vi "Build.vi"(9 "XYZTheta":dbl[](array[numeric]), 10 "Pattern Coordinates":dbl[][](array[numeric]), 11 "CAD Dispense in":refnum<class "CAD Dispense.lvclass">) -> (1 "Starting Coordinates":dbl[](array[numeric]), 3 "CAD Dispense out":refnum<class "CAD Dispense.lvclass">)   [LabVIEW 2016, in "CAD Dispense.lvclass"]
uses:
  CAD Dispense.lvclass
  CAD Dispense.lvclass/CAD Dispense.ctl
  <vilib>/Analysis/coordinate.llb/2D Cartesian Coordinate Rotation (Scalar).vi
  <vilib>/Analysis/NI_AALPro.lvlib
panel:
  out "Array 3":dbl[][](array[numeric])
  out "size(s) 2":i32
  out "size(s)":i32
  out "startXY,endXY":dbl[][](array[numeric])
  out "center portion":dbl[][](array[numeric])
  out "Array 2":dbl[][](array[numeric])
  out "Array":dbl[][](array[numeric])
  out "array w/ subset deleted 2":T1(array[cluster])
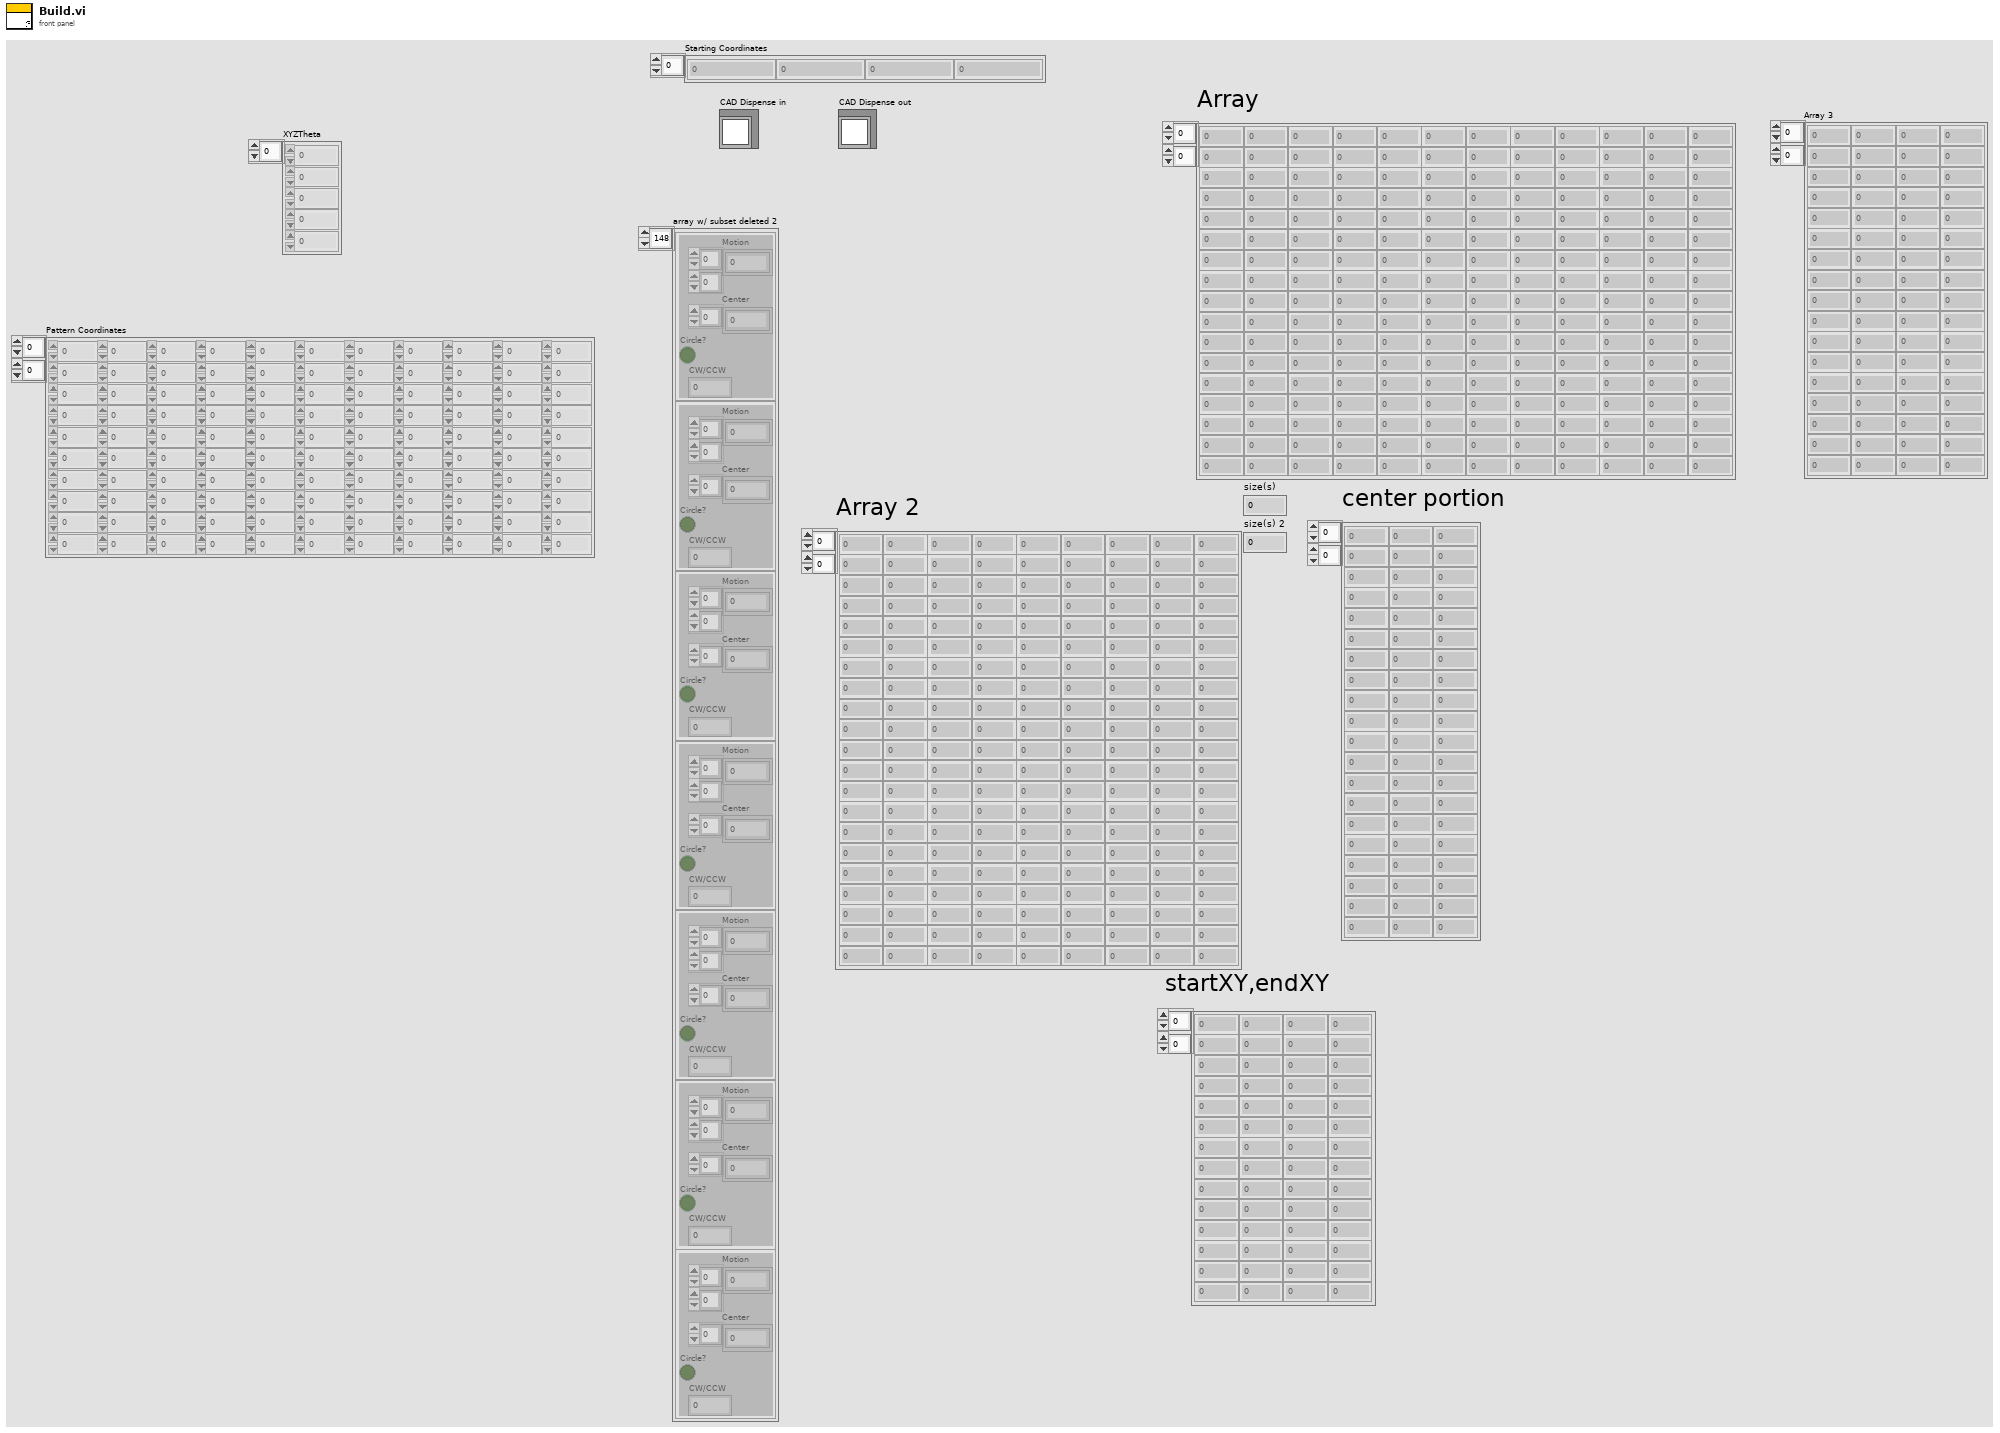
[diagram p1: front panel]
types:
  T1 = cluster{"Motion":dbl[][], "Center":dbl[], "Circle?":bool, "CW/CCW":dbl}[]
  T2 = cluster{"Motion":dbl[][], "Center":dbl[], "Circle?":bool, "CW/CCW":dbl}
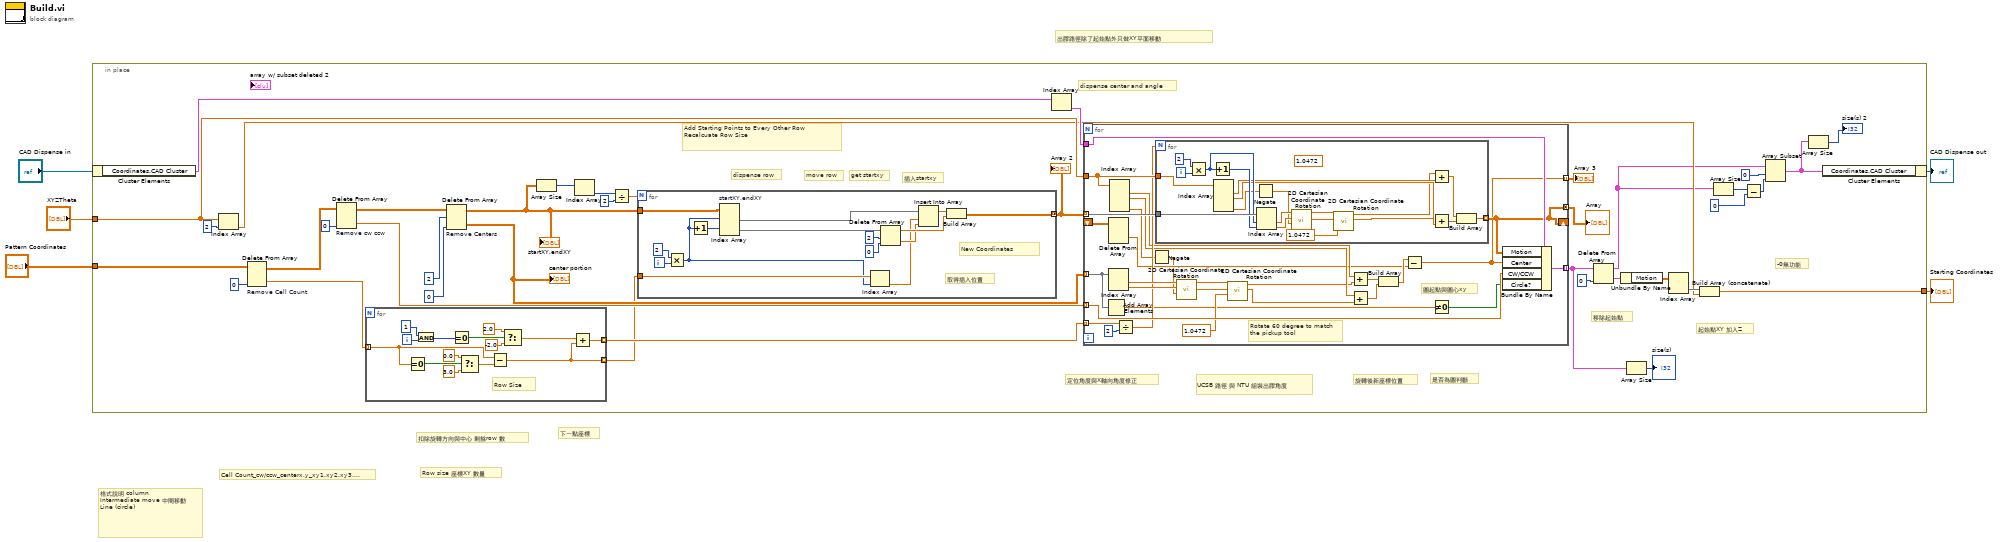
[diagram p0: block diagram]
diagram:
  # "出膠路徑除了起始點外只做XY平面移動"
  # "下一點座標"
  # "Cell Count_cw/ccw_centerx,y_xy1,xy2,xy3,..."
  # "格式說明 column\nIntermediate move 中間移動\nLine (circle)"
  # "扣除旋轉方向與中心 剩餘row 數"
  # "Row size 座標XY 數量"
  n1 = in-place {
    in-place-border: "XYZTheta" -> [w20]
    in-place-border: "Pattern Coordinates" -> [w31]
    in-place-border: [w17] -> w3
    # "-0無功能"
    # "起始點XY 加入Z"
    # "移除起始點"
    # "是否為圓判斷"
    # "旋轉後新座標位置"
    # "定位角度與X軸向角度修正"
    # "UCSB 路徑 與 NTU 組裝出膠角度"
    # "dispense center and angle"
    # "get startxy"
    # "dispense row"
    # "move row"
    # "插入startxy"
    # "Add Starting Points to Every Other Row\nRecalcuate Row Size"
    n2 = in-place-cluster #1("CAD Dispense in") -> ("Coordinates.CAD Cluster"=w33:T1)
    n3 = Index Array(array=w20, index=2) -> (element=w18:dbl)
    n4 = Delete From Array "Remove Cell Count"(array=w31, index (col)=0 ("disabled index (col)")) -> (deleted portion=w27:dbl[], array with subset deleted=w38:dbl[][])  [unwired: 2 in]
    n5 = Delete From Array "Remove cw ccw"(array=w38, index (col)=0 ("disabled index (col)")) -> (deleted portion=w43:dbl[], array with subset deleted=w39:dbl[][])  [unwired: 2 in]
    n6 = for {
      tunnel: w27 -> [w54] mode=indexing
      tunnel: [w46] -> w26 mode=indexing
      tunnel: [w45] -> w25 mode=indexing
      i -> [w47]
      # "Row Size"
      n7 = Equal To 0?(x=w54) -> (x = 0?=w55:bool)
      n8 = And(x=1, y=w47) -> (x .and. y?=w50:i32)
      n9 = Equal To 0?(x=w50) -> (x = 0?=w48:bool)
      n10 = Select(t=0.0, s=w55, f=3.0) -> (s? t:f=w58:dbl)
      n11 = Subtract(x=w54, y=w58) -> (x-y=w45:dbl)
      n12 = Select(t=2.0, s=w48, f=-2.0) -> (s? t:f=w51:dbl)
      n13 = Add(x=w51, y=w45) -> (x+y=w46:dbl)
    }
    n14 = Delete From Array "Remove Centers"(array=w39, length=2, index (col)=0 ("disabled index (col)")) -> (deleted portion=w44:dbl[][], array with subset deleted=w40:dbl[][])  [unwired: 1 in]
    "center portion" <- w44
    "startXY,endXY" <- w40
    n15 = Array Size(array=w40) -> (size(s)=w41:i32[])
    n16 = Index Array(array=w41) -> (element=w30:i32)  [unwired: 1 in]
    n17 = Divide(x=w30, y=2) -> (x/y=w28:dbl)
    n18 = for {
      N: w28 -> [_]
      tunnel: w40 -> [w122]
      tunnel: [w114] -> w42 mode=concatenating
      tunnel: w25 -> [w109]
      i -> [w115]
      # "取得插入位置"
      # "New Coordinates"
      n19 = Multiply(x=2, y=w115) -> (x*y=w108:i32)
      n20 = Increment(x=w108) -> (x+1=w110:i32)
      n21 = Index Array "startXY,endXY"(array=w122, index (row) #1=w108, index (row) #2=w110) -> (element #1=w118:dbl[], element #2=w120:dbl[])  [unwired: 2 in]
      n22 = Index Array(array=w109, index=w108) -> (element=w111:dbl)
      n23 = Delete From Array(array=w120, length=2, index=0) -> (deleted portion=w112:dbl[], array with subset deleted=w116:dbl[])
      n24 = Insert Into Array(array=w118, index=w111, new element=w112) -> (w117:dbl[])
      n25 = Build Array(w117, w116) -> (w114:dbl[][])
    }
    "Array 2" <- w42
    n26 = Index Array(array=w33) -> (element=w32:T2)  [unwired: 1 in]
    n27 = for {
      tunnel: w26 -> [w85] mode=indexing
      tunnel: w42 -> [w80] mode=indexing
      tunnel: w43 -> [w83] mode=indexing
      tunnel: w44 -> [w79] mode=indexing
      tunnel: w20 -> [w86]
      tunnel: w32 -> [w84]
      tunnel: [w81] -> w11 mode=indexing
      shift-right: [w60] -> _
      shift-left: _ -> [w70]
      tunnel: [w60] -> w7 mode=concatenating
      tunnel: [w59] -> w6 mode=indexing
      # "圓起點與圓心xy"
      # "Rotate 60 degree to match the pickup tool"
      n28 = Add Array Elements(numeric array=w79) -> (sum=w61:dbl)
      n29 = Delete From Array(array=w70) -> (deleted portion=w69:dbl[])  [unwired: 3 in, 1 out]
      n30 = Index Array(array=w79) -> (element #1=w78:dbl, element #2=w77:dbl)  [unwired: 2 in]
      n31 = Index Array(array=w86) -> (element #1=w75:dbl, element #2=w72:dbl, element #4=w68:dbl)  [unwired: 4 in, 1 out]
      n32 = Divide(x=w85, y=2) -> (x/y=w76:dbl)
      n33 = Negate(x=w68) -> (-x=w67:dbl)
      n34 = for {
        N: w76 -> [_]
        tunnel: w80 -> [w107]
        tunnel: [w95] -> w60 mode=indexing
        tunnel: w86 -> [w103]
        i -> [w96]
        (unwired) 1.0472 ("theta")
        n35 = Multiply(x=2, y=w96) -> (x*y=w105:i32)
        n36 = Increment(x=w105) -> (x+1=w104:i32)
        n37 = Index Array(array=w103) -> (element #1=w98:dbl, element #2=w97:dbl, element #4=w94:dbl)  [unwired: 4 in, 1 out]
        n38 = Negate(x=w94) -> (-x=w93:dbl)
        n39 = Index Array(array=w107, index #1=w105, index #2=w104) -> (element #1=w100:dbl, element #2=w99:dbl)
        n40 = call-poly <vilib>:"2D Cartesian Coordinate Rotation.vi"("theta"=w93, "y"=w99, "x"=w100) -> ("y out"=w91:dbl, "x out"=w92:dbl)  [unwired: 6 in, 1 out]
        n41 = call-poly <vilib>:"2D Cartesian Coordinate Rotation.vi"("theta"=1.0472, "y"=w91, "x"=w92) -> ("y out"=w89:dbl, "x out"=w90:dbl)  [unwired: 6 in, 1 out]
        n42 = Add(x=w90, y=w98) -> (x+y=w102:dbl)
        n43 = Add(x=w89, y=w97) -> (x+y=w101:dbl)
        n44 = Build Array(w102, w101) -> (w95:dbl[])
      }
      n45 = call-poly <vilib>:"2D Cartesian Coordinate Rotation.vi"("theta"=w67, "y"=w77, "x"=w78) -> ("y out"=w65:dbl, "x out"=w66:dbl)  [unwired: 6 in, 1 out]
      n46 = call-poly <vilib>:"2D Cartesian Coordinate Rotation.vi"("theta"=1.0472, "y"=w65, "x"=w66) -> ("y out"=w62:dbl, "x out"=w63:dbl)  [unwired: 6 in, 1 out]
      n47 = Add(x=w75, y=w63) -> (x+y=w74:dbl)
      n48 = Add(x=w72, y=w62) -> (x+y=w73:dbl)
      n49 = Build Array(w74, w73) -> (w71:dbl[])
      n50 = Subtract(x=w71, y=w69) -> (x-y=w59:dbl[])
      n51 = Not Equal To 0?(x=w61) -> (x != 0?=w82:bool)
      n52 = Bundle By Name(cluster=w84, "Motion"=w60, "Center"=w59, "CW/CCW"=w83, "Circle?"=w82) -> (w81:T2)
    }
    "Array" <- w7
    "Array 3" <- w6
    n53 = Delete From Array(array=w11, index=0) -> (deleted portion=w24:T2, array with subset deleted=w16:T1)  [unwired: 1 in]
    n54 = Unbundle By Name(w24) -> ("Motion"=w22:dbl[][])
    n55 = Array Size(array=w11) -> (size(s)=→"size(s)":i32)
    n56 = Index Array(array=w22) -> (element=w21:dbl[])  [unwired: 2 in]
    n57 = Build Array (concatenate)(w21, w18) -> (w17:dbl[])
    n58 = Array Size(array=w16) -> (size(s)=w14:i32)
    n59 = Subtract(x=w14, y=0) -> (x-y=w12:i32)
    n60 = Array Subset(array=w16, index=0, length=w12) -> (w9:T1)
    n61 = Array Size(array=w9) -> (size(s)=→"size(s) 2":i32)
    n62 = in-place-cluster #1("Coordinates.CAD Cluster"=w9) -> (→"CAD Dispense out":refnum<class "CAD Dispense.lvclass">)
  }
  "Starting Coordinates" <- w3
